vi "Asserts.vi"(0 "VI Reference In":refnum<vi>, 1 "Label (VI Title)":string="Default", 11 "error in (no error)":errorcluster) -> (4 "VI Reference Out":refnum<vi>, 15 "error out":errorcluster)   [LabVIEW 2016, in "DronaTest.lvlib"]
uses:
  DronaTest.lvlib
  <vilib>/addons/_JKI Toolkits/Caraya/classes/Test/Test.lvclass
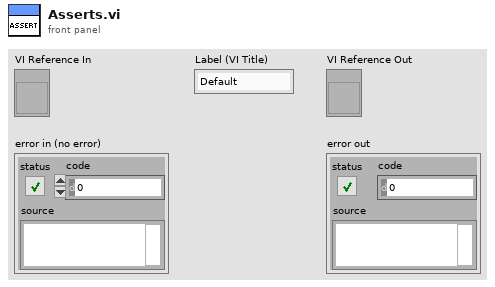
[diagram p1: front panel]
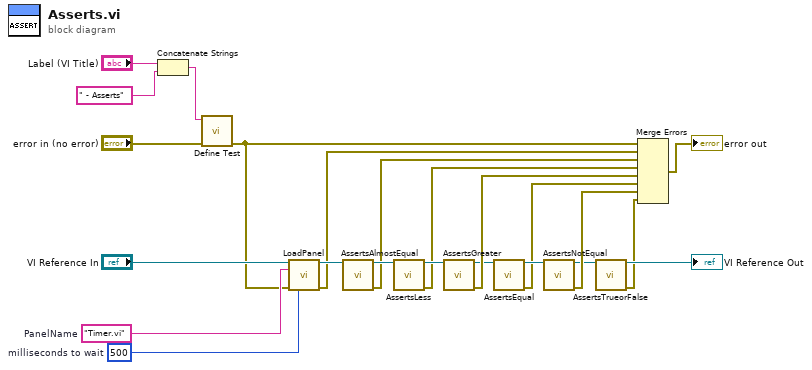
[diagram p0: block diagram]
diagram:
  w16 = u32 500  # milliseconds to wait
  w17 = "Timer.vi"  # PanelName
  n1 = Concatenate Strings("Label (VI Title)", " - Asserts" ("Label (VI Title)")) -> (w19:string)
  n2 = call <vilib>:"Define Test.vi"("error in (no error)"="error in (no error)", "Label (VI Title)"=w19) -> ("error out"=w15:errorcluster)  [unwired: 9 in]
  n3 = call "LoadPanel.vi"("VI in"="VI Reference In", "Panel Name"=w17, "error in (no error)"=w15, "milliseconds to wait"=w16) -> ("VI out"=w14:refnum<vi>, "error out"=w11:errorcluster)  [unwired: 10 in]
  n4 = call "AssertsAlmostEqual.vi"("VI Reference In"=w14) -> ("VI Reference Out"=w13:refnum<vi>, "error out"=w10:errorcluster)  [unwired: 13 in]
  n5 = call "AssertsLess.vi"("VI Reference In"=w13) -> ("VI Reference Out"=w12:refnum<vi>, "error out"=w9:errorcluster)  [unwired: 13 in]
  n6 = call "AssertsGreater.vi"("VI Reference In"=w12) -> ("VI Reference Out"=w6:refnum<vi>, "error out"=w8:errorcluster)  [unwired: 13 in]
  n7 = call "AssertsEqual.vi"("VI Reference In"=w6) -> ("VI Reference Out"=w7:refnum<vi>, "error out"=w5:errorcluster)  [unwired: 13 in]
  n8 = call "AssertsNotEqual.vi"("VI Reference In"=w7) -> ("VI Reference Out"=w3:refnum<vi>, "error out"=w4:errorcluster)  [unwired: 13 in]
  n9 = call "AssertsTrueorFalse.vi"("VI Reference In"=w3) -> ("VI Reference Out"=→"VI Reference Out":refnum<vi>, "error out"=w1:errorcluster)  [unwired: 13 in]
  n10 = Merge Errors(w15, w11, w10, w9, w8, w5, w4, w1) -> (→"error out":errorcluster)
